vi "getDecimalSeparatorString.vi"(10 "Decimal Separator":T1, 11 "StringFormatter":refnum<class "StringFormatter.lvclass">) -> (2 "Formatter String":string)   [LabVIEW 2013, in "OpenStringFormatter.lvlib" / "StringFormatter.lvclass"]
uses:
  StringFormatter.lvclass
  Localization Decimal Separator -- enum.ctl
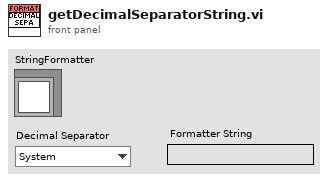
[diagram p1: front panel]
types:
  T1 = typedef "OpenStringFormatter.lvlib/StringFormatter.lvclass/Localization Decimal Separator -- enum.ctl" = enum16{"System", "Comma", "Dot"}
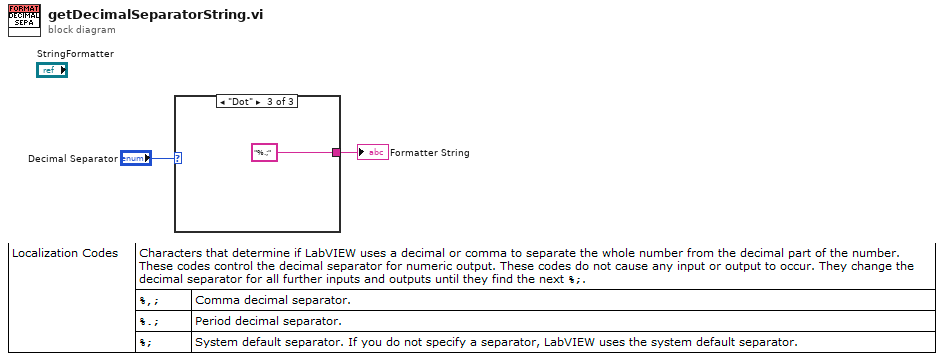
[diagram p0: block diagram]
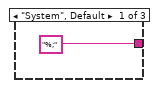
[diagram p2: hidden frame]
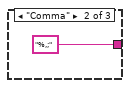
[diagram p3: hidden frame]
diagram:
  n1 = case shown="\"Dot\"" "Decimal Separator" {
    tunnel: ["%;" "%,;" "%.;"] -> w1
    frame "System", Default {
    }
    frame "Comma" {
    }
    frame "Dot" {
    }
  }
  "Formatter String" <- w1
